vi "LCD with custom commands_Project.vi"() -> ()   [LabVIEW 2014]
uses:
  <vilib>/MakerHub/LINX/Public/Utilities/Open Serial.vi
  <vilib>/MakerHub/LINX/LMH-LINX.lvlib
panel:
  in  "Animation":bool
  in  "Line 3":string
  in  "Line 2":string
  in  "Line 1":string
  in  "Line 0":string
  in  "Stop button":bool caption="Stop"
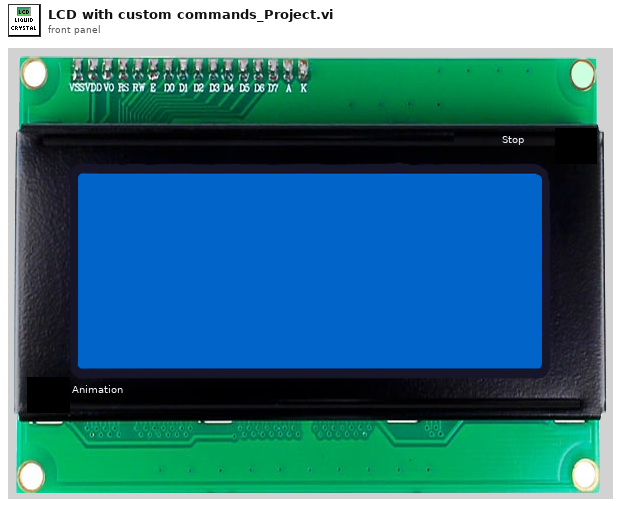
[diagram p1: front panel]
types:
  T1 = typedef "LMH-LINX.lvlib/LINX Ref.ctl" = cluster{"IO":T2, "Interface":T3, "LINX Device Config":T4}
  T2 = typedef "LMH-LINX.lvlib/Platform.ctl" = enum16{"Remote", "Local"}
  T3 = typedef "LMH-LINX.lvlib/Interface.ctl" = enum16{"Serial", "TCP"}
  T4 = typedef "LMH-LINX.lvlib/Device.lvlib/LINX Device Config.ctl" = cluster{"Interface":T3, "COM Port":refnum<visa-resource-name>, "TCP Configuration":T5, "Device Family":u8, "Device ID":u8, "Device Name":string, "TCP Ref":refnum<k5>, "Channels":T6}
  T5 = typedef "LMH-LINX.lvlib/Device.lvlib/TCP Config.ctl" = cluster{"IP Address":string, "Port":u16}
  T6 = typedef "LMH-LINX.lvlib/Channels.ctl" = cluster{"DI":u8[], "DO":u8[], "AI":u8[], "AO":u8[], "PWM":u8[], "QE":u8[], "UART":u8[], "I2C 2":u8[], "SPI":u8[], "CAN":u8[], "Servo":u8[], "AI Ref (V)":dbl, "AI Resolution (Bits)":u8, "AO Ref (V)":dbl, "AO Resolution (Bits)":u8}
  T7 = enum8{"Enabled", "Disabled", "Disabled and Grayed Out"}
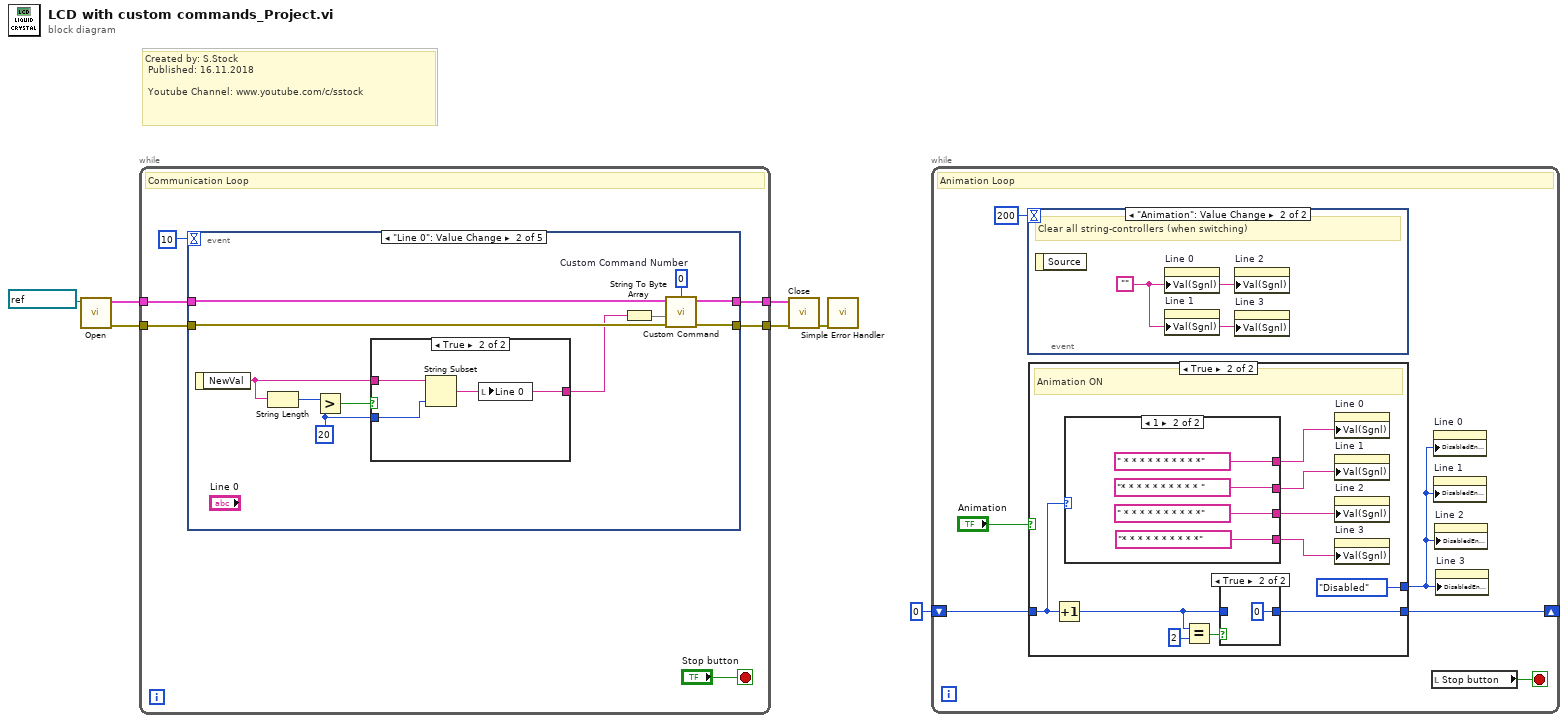
[diagram p0: block diagram]
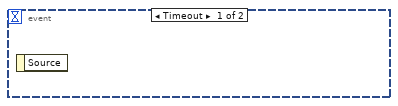
[diagram p2: hidden frame]
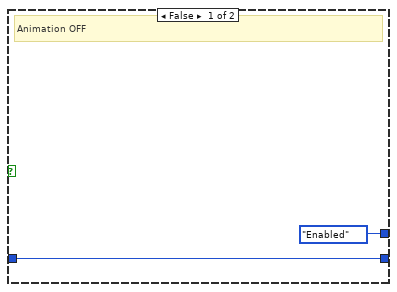
[diagram p3: hidden frame]
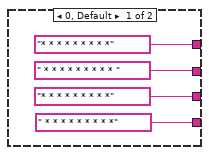
[diagram p4: hidden frame]
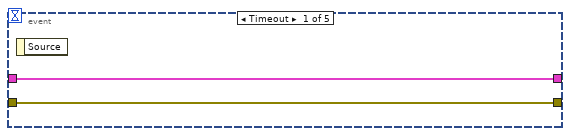
[diagram p6: hidden frame]
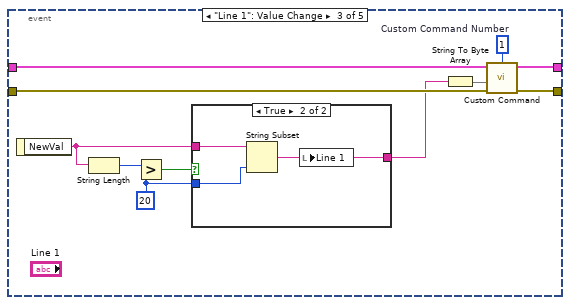
[diagram p8: hidden frame]
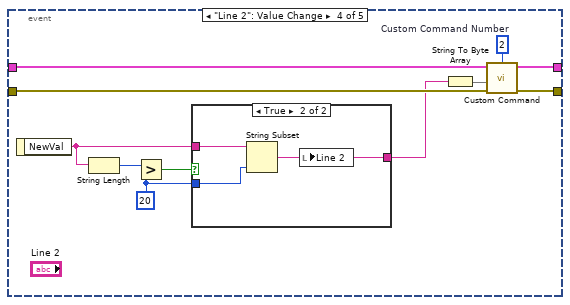
[diagram p10: hidden frame]
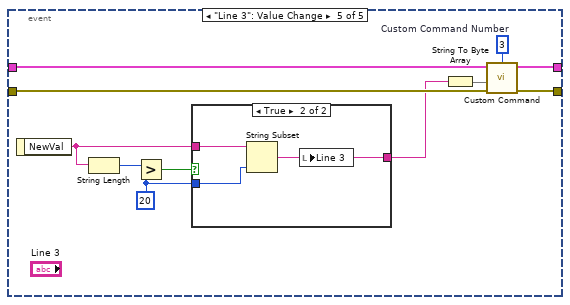
[diagram p12: hidden frame]
diagram:
  # "Created by: S.Stock\n Published: 16.11.2018\n\n Youtube Channel: www.youtube.com/c/sstock"
  n1 = call-poly <vilib>:"Open.vi"("Serial Port"=refnum<visa-resource-name> "COM10") -> ("Error Out"=w5:errorcluster, "LINX Resource"=w6:T1)  [unwired: 8 in, 1 out]
  n2 = while {
    tunnel: w6 -> [w13]
    tunnel: w5 -> [w12]
    tunnel: [w10] -> w3
    tunnel: [w9] -> w2
    stop <- "Stop button" stop-if-true
    # "Communication Loop"
    n3 = event shown="[1] \"Line 0\": Value Change" {
      selector: _ -> [_ _ _ _ _]
      dyn-events: _ -> [_ _ _ _ _]
      timeout: 10 -> [_ _ _ _ _]
      tunnel: w13 -> [w15 w22 w37 w52 w67]
      tunnel: [w15 w20 w35 w50 w65] -> w10
      tunnel: [w14 w19 w34 w49 w64] -> w9
      tunnel: w12 -> [w14 w21 w36 w51 w66]
      event Timeout {
        n4 = event-data() -> ()  [unwired: 1 in, 1 out]
      }
      event "Line 0": Value Change {
        w16 = u16 0  # Custom Command Number
        w23 = 20 ("y")
        n5 = event-data() -> ("NewVal"=w24:string)  [unwired: 1 in]
        n6 = String Length(string=w24) -> (length=w26:i32)
        n7 = Greater?(x=w26, y=w23) -> (0:w25:bool)
        n8 = case shown="True" w25 {
          tunnel: w24 -> [w27 w30]
          tunnel: w23 -> [_ w29]
          tunnel: [w27 w28] -> w17
          frame False {
          }
          frame True {
            n9 = String Subset(string=w30, length (rest)=w29) -> (substring=w28:string)  [unwired: 1 in]
            n10 = local write "Line 0"(w28) -> ()
          }
        }
        n11 = String To Byte Array(string=w17) -> (unsigned byte array=w18:u8[])
        n12 = call <vilib>:"Custom Command.vi"("Error In"=w21, "Data"=w18, "Custom Command Number"=w16, "LINX Resource"=w22) -> ("Error Out"=w19:errorcluster, "LINX Resource"=w20:T1)  [unwired: 4 in, 2 out]
      }
      event "Line 1": Value Change {
        w31 = u16 1  # Custom Command Number
        w38 = 20 ("y")
        n13 = event-data() -> ("NewVal"=w39:string)  [unwired: 1 in]
        n14 = String Length(string=w39) -> (length=w41:i32)
        n15 = Greater?(x=w41, y=w38) -> (0:w40:bool)
        n16 = case shown="True" w40 {
          tunnel: w39 -> [w42 w45]
          tunnel: w38 -> [_ w44]
          tunnel: [w42 w43] -> w32
          frame False {
          }
          frame True {
            n17 = String Subset(string=w45, length (rest)=w44) -> (substring=w43:string)  [unwired: 1 in]
            n18 = local write "Line 1"(w43) -> ()
          }
        }
        n19 = String To Byte Array(string=w32) -> (unsigned byte array=w33:u8[])
        n20 = call <vilib>:"Custom Command.vi"("Error In"=w36, "Data"=w33, "Custom Command Number"=w31, "LINX Resource"=w37) -> ("Error Out"=w34:errorcluster, "LINX Resource"=w35:T1)  [unwired: 4 in, 2 out]
      }
      event "Line 2": Value Change {
        w46 = u16 2  # Custom Command Number
        w53 = 20 ("y")
        n21 = event-data() -> ("NewVal"=w54:string)  [unwired: 1 in]
        n22 = String Length(string=w54) -> (length=w56:i32)
        n23 = Greater?(x=w56, y=w53) -> (0:w55:bool)
        n24 = case shown="True" w55 {
          tunnel: w54 -> [w57 w60]
          tunnel: w53 -> [_ w59]
          tunnel: [w57 w58] -> w47
          frame False {
          }
          frame True {
            n25 = String Subset(string=w60, length (rest)=w59) -> (substring=w58:string)  [unwired: 1 in]
            n26 = local write "Line 2"(w58) -> ()
          }
        }
        n27 = String To Byte Array(string=w47) -> (unsigned byte array=w48:u8[])
        n28 = call <vilib>:"Custom Command.vi"("Error In"=w51, "Data"=w48, "Custom Command Number"=w46, "LINX Resource"=w52) -> ("Error Out"=w49:errorcluster, "LINX Resource"=w50:T1)  [unwired: 4 in, 2 out]
      }
      event "Line 3": Value Change {
        w61 = u16 3  # Custom Command Number
        w68 = 20 ("y")
        n29 = event-data() -> ("NewVal"=w69:string)  [unwired: 1 in]
        n30 = String Length(string=w69) -> (length=w71:i32)
        n31 = Greater?(x=w71, y=w68) -> (0:w70:bool)
        n32 = case shown="True" w70 {
          tunnel: w69 -> [w72 w75]
          tunnel: w68 -> [_ w74]
          tunnel: [w72 w73] -> w62
          frame False {
          }
          frame True {
            n33 = String Subset(string=w75, length (rest)=w74) -> (substring=w73:string)  [unwired: 1 in]
            n34 = local write "Line 3"(w73) -> ()
          }
        }
        n35 = String To Byte Array(string=w62) -> (unsigned byte array=w63:u8[])
        n36 = call <vilib>:"Custom Command.vi"("Error In"=w66, "Data"=w63, "Custom Command Number"=w61, "LINX Resource"=w67) -> ("Error Out"=w64:errorcluster, "LINX Resource"=w65:T1)  [unwired: 4 in, 2 out]
      }
    }
  }
  n37 = call <vilib>:"Close.vi"("Error In"=w2, "LINX Resource"=w3) -> ("Error Out"=w4:errorcluster)  [unwired: 9 in]
  n38 = call <vilib>:"Simple Error Handler.vi"("error in (no error)"=w4) -> ()  [unwired: 4 in, 5 out]
  n39 = while {
    shift-right: [w80] -> _
    shift-left: 0 -> [w81]
    stop <- w76 stop-if-true
    # "Animation Loop"
    n40 = event shown="[1] \"Animation\": Value Change" {
      selector: _ -> [_ _]
      dyn-events: _ -> [_ _]
      timeout: 200 -> [_ _]
      event Timeout {
        n41 = event-data() -> ()  [unwired: 1 in, 1 out]
      }
      event "Animation": Value Change {
        w82 = ""
        # "Clear all string-controllers (when switching)"
        n42 = event-data() -> ()  [unwired: 1 in, 1 out]
        n43 = property on="Line 0" class="Str"("Val(Sgnl)"=w82) -> ()  [unwired: 2 in, 2 out]
        n44 = property on="Line 1" class="Str"("Val(Sgnl)"=w82) -> ()  [unwired: 2 in, 2 out]
        n45 = property on="Line 2" class="Str"("Val(Sgnl)"=w82) -> ()  [unwired: 2 in, 2 out]
        n46 = property on="Line 3" class="Str"("Val(Sgnl)"=w82) -> ()  [unwired: 2 in, 2 out]
      }
    }
    n47 = case shown="True" "Animation" {
      tunnel: w81 -> [w84 w94]
      tunnel: [w84 w93] -> w80
      tunnel: [T7."Enabled" ("Disabled") T7."Disabled" ("Disabled")] -> w79
      frame False {
        # "Animation OFF"
      }
      frame True {
        # "Animation ON"
        n48 = Increment(x=w94) -> (x+1=w90:i32)
        n49 = case shown="1" w94 {
          tunnel: ["* * * * * * * * *" " * * * * * * * * * *"] -> w88
          tunnel: [" * * * * * * * * * " "* * * * * * * * * * "] -> w87
          tunnel: ["* * * * * * * * *" " * * * * * * * * * *"] -> w86
          tunnel: [" * * * * * * * * *" "* * * * * * * * * *"] -> w85
          frame 0, Default {
          }
          frame 1 {
          }
        }
        n50 = Equal?(x=w90, y=2) -> (x = y?=w91:bool)
        n51 = case shown="True" w91 {
          tunnel: [w103 0] -> w93
          tunnel: w90 -> [w103 _]
          frame False {
          }
          frame True {
          }
        }
        n52 = property on="Line 0" class="Str"("Val(Sgnl)"=w88) -> ()  [unwired: 2 in, 2 out]
        n53 = property on="Line 1" class="Str"("Val(Sgnl)"=w87) -> ()  [unwired: 2 in, 2 out]
        n54 = property on="Line 2" class="Str"("Val(Sgnl)"=w86) -> ()  [unwired: 2 in, 2 out]
        n55 = property on="Line 3" class="Str"("Val(Sgnl)"=w85) -> ()  [unwired: 2 in, 2 out]
      }
    }
    n56 = local read "Stop button"() -> (w76:bool)
    n57 = property on="Line 0" class="Str"("DisabledEnum"=w79) -> ()  [unwired: 2 in, 2 out]
    n58 = property on="Line 1" class="Str"("DisabledEnum"=w79) -> ()  [unwired: 2 in, 2 out]
    n59 = property on="Line 2" class="Str"("DisabledEnum"=w79) -> ()  [unwired: 2 in, 2 out]
    n60 = property on="Line 3" class="Str"("DisabledEnum"=w79) -> ()  [unwired: 2 in, 2 out]
  }
